vi "get_item_by_name.vi"(8 "error in (no error)":errorcluster, 10 "item_name":string, 11 "Table in":refnum<class "Table.lvclass">) -> (0 "error out":errorcluster, 1 "Item":refnum<class "Item.lvclass">, 3 "Table out":refnum<class "Table.lvclass">)   [LabVIEW 2020, in "toml_edit.lvlib" / "Table.lvclass"]
uses:
  Table.lvclass
  Item/Item.lvclass
  Table.lvclass/Table.ctl
  Item/type--enum.ctl
  dragon_toml_64.dll
panel:
  out "item_type":T1
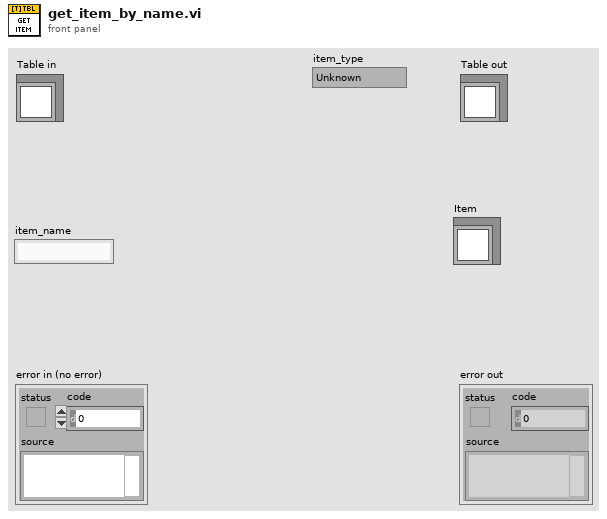
[diagram p1: front panel]
types:
  T1 = typedef "toml_edit.lvlib/Item.lvclass/type--enum.ctl" = enum16{"Unknown", "None", "Value", "ArrayOfTables", "Table"}
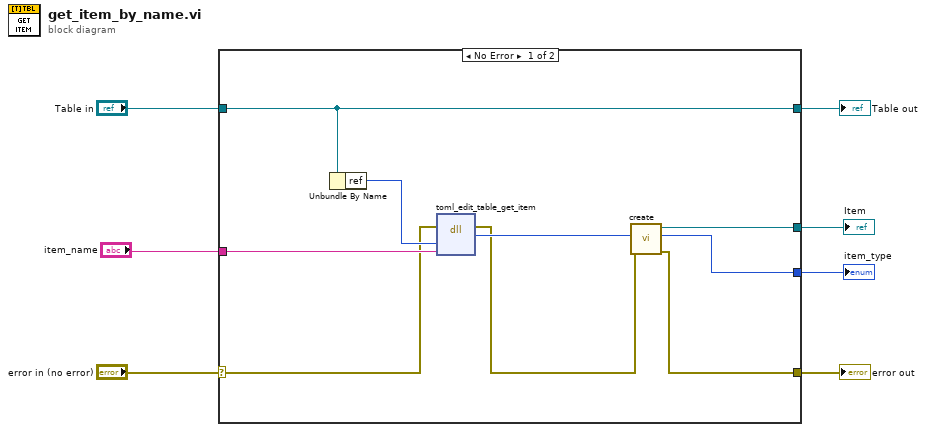
[diagram p0: block diagram]
diagram:
  n1 = case shown="No Error" "error in (no error)" {
    selector: "error in (no error)" -> [w13 w18]
    tunnel: [w9 w18] -> w6
    tunnel: [w11 w17] -> w4
    tunnel: "Table in" -> [w11 w17]
    tunnel: "item_name" -> [w14 _]
    tunnel: [w10 _] -> w2
    tunnel: [w8 _] -> w1
    frame No Error {
      n2 = Unbundle By Name(w11) -> ("ref"=w15:u64)
      n3 = dll-call lib="C:/Projects/labview-project-load-tools/source/submodules/toml-edit-labview/lv_src/dragon_toml_*.*" fn="toml_edit_table_get_item"(error in=w13, "table_ref"=w15, "item_name"=w14) -> (error out=w12:errorcluster, "item_ref"=w16:u64)  [unwired: 4 in, 1 out]
      n4 = call "create.vi"("error in (no error)"=w12, "ref"=w16) -> ("error out"=w9:errorcluster, "item_type"=w8:T1, "Item out"=w10:refnum<class "Item.lvclass">)  [unwired: 7 in]
    }
    frame Error {
    }
  }
  "error out" <- w6
  "Table out" <- w4
  "Item" <- w2
  "item_type" <- w1
